vi "Configure.vi"(8 "error in (no error)":errorcluster, 11 "DemoCamera in":refnum<class "DemoCamera.lvclass">) -> (0 "error out":errorcluster, 3 "DemoCamera out":refnum<class "DemoCamera.lvclass">)   [LabVIEW 2020, in "DemoCamera.lvlib" / "DemoCamera.lvclass"]
uses:
  DemoCamera.lvclass
  Hardware Abstraction Layer/Component/Camera/Camera/Camera.lvclass
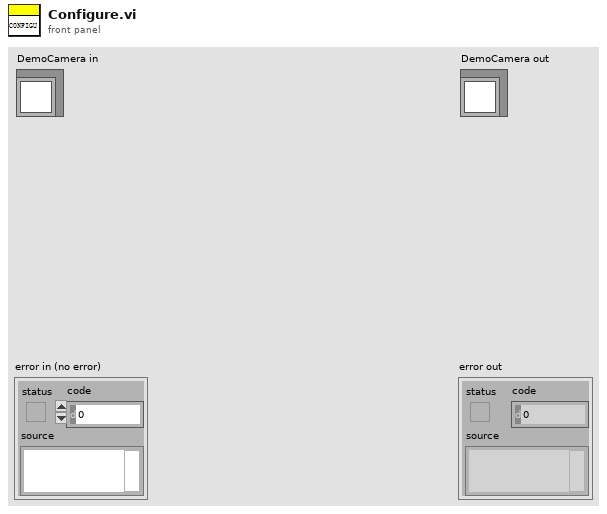
[diagram p1: front panel]
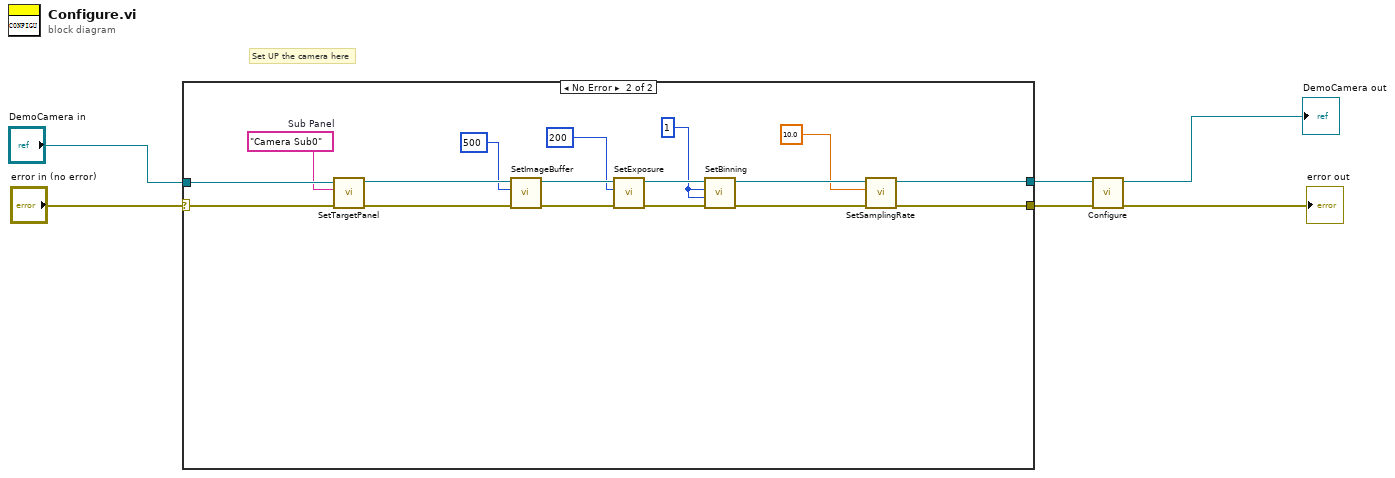
[diagram p0: block diagram]
diagram:
  # "Set UP the camera here"
  n1 = case shown="No Error" "error in (no error)" {
    selector: "error in (no error)" -> [w8 w23]
    tunnel: [w8 w12] -> w4
    tunnel: "DemoCamera in" -> [w7 w25]
    tunnel: [w7 w10] -> w2
    frame Error {
    }
    frame No Error {
      w13 = 1 ("Setting.Binning.BinX")
      w24 = "Camera Sub0"  # Sub Panel
      n2 = call-dynamic "SetTargetPanel.vi"("error in (no error)"=w23, "TargetPanel"=w24, "GRMActor in"=w25) -> ("error out"=w22:errorcluster, "GRMActor out"=w20:refnum<class "DemoCamera.lvclass">)  [unwired: 7 in]
      n3 = call-dynamic "SetImageBuffer.vi"("error in (no error)"=w22, "max queue size (-1, unlimited)"=500, "Camera in"=w20) -> ("error out"=w21:errorcluster, "Camera out"=w17:refnum<class "DemoCamera.lvclass">)  [unwired: 7 in]
      n4 = call-dynamic "SetExposure.vi"("error in (no error)"=w21, "Setting.Exposure"=200, "DemoCamera in"=w17) -> ("error out"=w18:errorcluster, "DemoCamera out"=w14:refnum<class "DemoCamera.lvclass">)  [unwired: 7 in]
      n5 = call-dynamic "SetBinning.vi"("error in (no error)"=w18, "Setting.Binning.BinY"=w13, "Setting.Binning.BinX"=w13, "Camera in"=w14) -> ("error out"=w15:errorcluster, "Camera out"=w11:refnum<class "DemoCamera.lvclass">)  [unwired: 6 in]
      n6 = call-dynamic "SetSamplingRate.vi"("error in (no error)"=w15, "SamplingRate(Hz)"=10.0, "Device in"=w11) -> ("error out"=w12:errorcluster, "Device out"=w10:refnum<class "DemoCamera.lvclass">)  [unwired: 7 in]
    }
  }
  n7 = call-parent "Configure.vi"("error in (no error)"=w4, "GRMActor in"=w2) -> ("error out"=→"error out":errorcluster, "GRMActor out"=→"DemoCamera out":refnum<class "DemoCamera.lvclass">)  [unwired: 8 in]
